vi "Get Sample Rate.vi"(8 "error in (no error)":errorcluster, 11 "RTL-SDR in":refnum<class "RTL-SDR.lvclass">) -> (0 "error out":errorcluster, 2 "Sample Rate (Hz)":u32, 3 "RTL-SDR out":refnum<class "RTL-SDR.lvclass">)   [LabVIEW 2015, in "RTL-SDR.lvclass"]
doc: "Created IvanLis by LabVIEW Portal\nProfile: http://labviewportal.org/memberlist.php?mode=viewprofile&u=987\neMail: IvanLisanov@gMail.com\nTelegram: https://t.me/IvanLis"
uses:
  RTL-SDR.lvclass
  RTL-SDR.lvclass/RTL-SDR.ctl
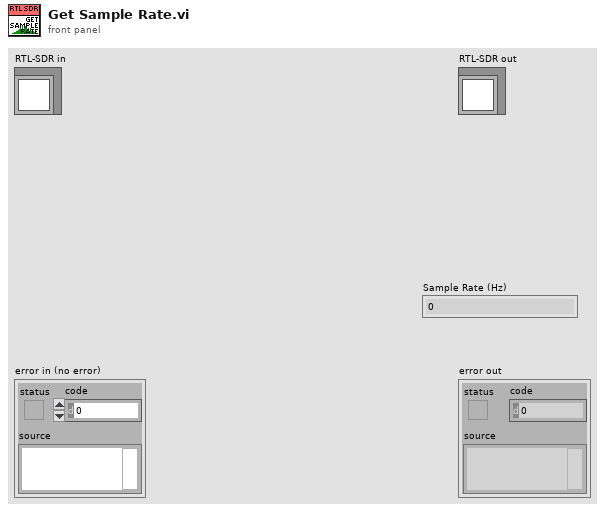
[diagram p1: front panel]
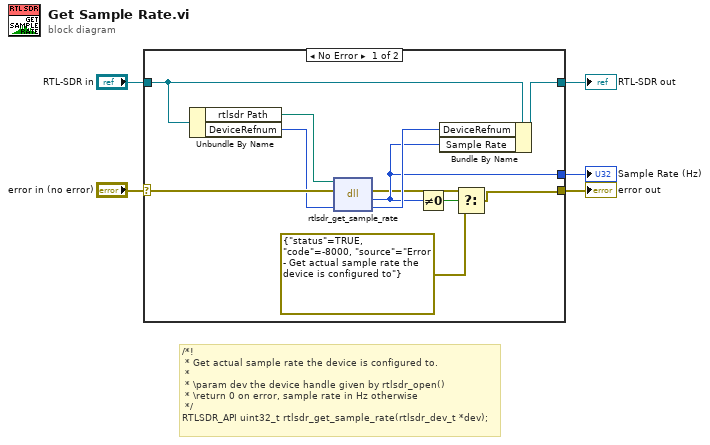
[diagram p0: block diagram]
diagram:
  # "/*!\n * Get actual sample rate the device is configured to.\n *\n * \\param dev the device handle given by rtlsdr_open()\n * \\return 0 on error, sample rate in Hz otherwise\n */\nRTLSDR_API uint32_t rtlsdr_get_sample_rate(rtlsdr_dev_t *dev);"
  n1 = case shown="No Error" "error in (no error)" {
    selector: "error in (no error)" -> [w16 w18]
    tunnel: [w6 w18] -> w4
    tunnel: [w12 w17] -> w2
    tunnel: "RTL-SDR in" -> [w15 w17]
    tunnel: [w8 _] -> w1
    frame No Error {
      n2 = Unbundle By Name(w15) -> ("rtlsdr Path"=w14:path, "DeviceRefnum"=w13:u64)
      n3 = dll-call lib="C:/Users/Ivan/Desktop/D-23-09-24 (RTL-SDR)/Project (Pelleng-SDR)/RTL-SDR Class/dll/rtlsdr.*" fn="rtlsdr_get_sample_rate"(path in=w14, error in=w16, "DeviceRefnum"=w13) -> (error out=w7:errorcluster, "return type"=w8:u32, "DeviceRefnum"=w11:u64)  [unwired: 1 in, 1 out]
      n4 = Not Equal To 0?(x=w8) -> (x != 0?=w10:bool)
      n5 = Bundle By Name(cluster=w15, "DeviceRefnum"=w11, "Sample Rate"=w8) -> (w12:refnum<class "RTL-SDR.lvclass">)
      n6 = Select(t=w7, s=w10, f=errorcluster {"status"=TRUE, "code"=-8000, "source"="Error - Get actual sample rate the device is configured to"} ("error out")) -> (s? t:f=w6:errorcluster)
    }
    frame Error {
    }
  }
  "error out" <- w4
  "RTL-SDR out" <- w2
  "Sample Rate (Hz)" <- w1
